vi "MailWake.vi"() -> ()   [LabVIEW 2012]
panel:
  out "Messages:":string[][](table)
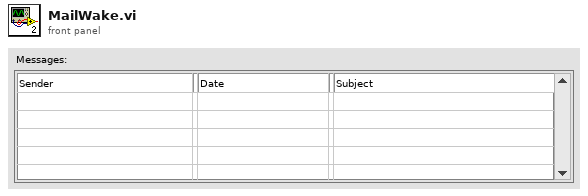
[diagram p1: front panel]
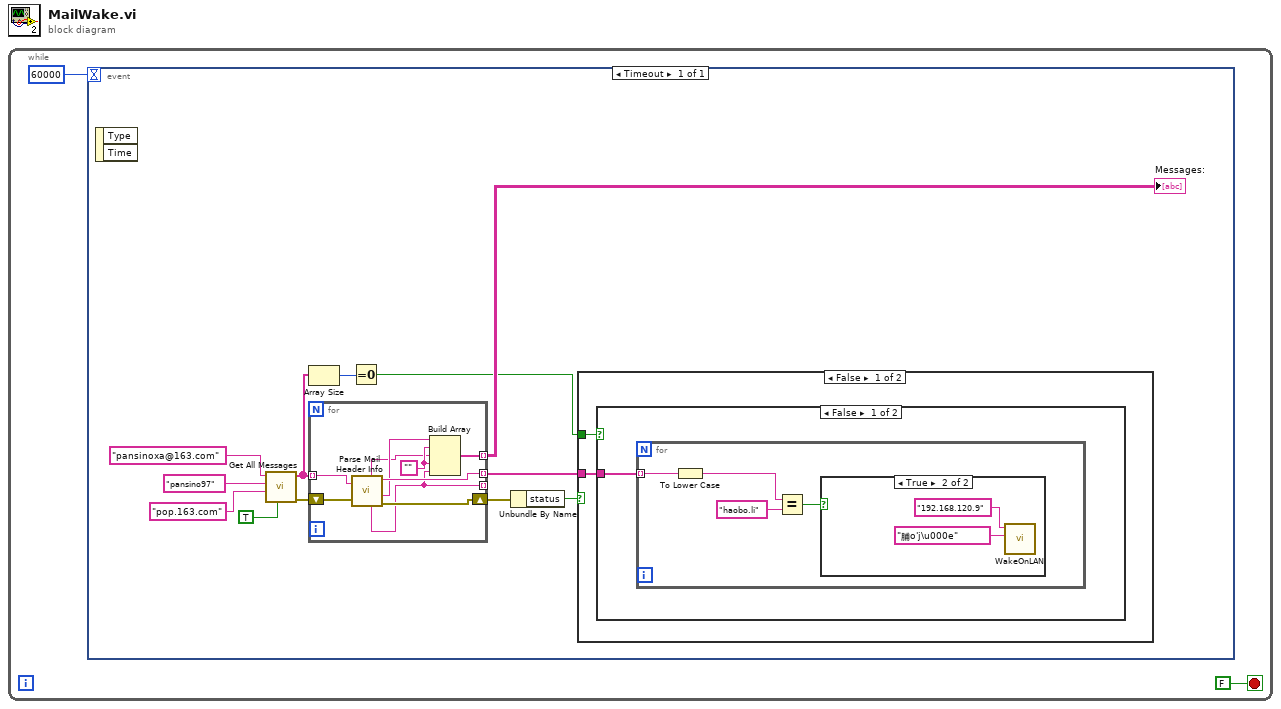
[diagram p0: block diagram]
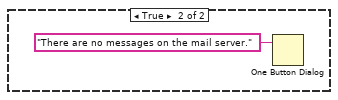
[diagram p3: hidden frame]
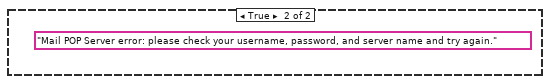
[diagram p4: hidden frame]
diagram:
  n1 = while {
    stop <- FALSE stop-if-true
    n2 = event shown="[0] Timeout" {
      selector: _ -> [_]
      dyn-events: _ -> [_]
      timeout: 60000 -> [_]
      event Timeout {
        n3 = event-data() -> ()  [unwired: 1 in, 2 out]
        n4 = call "Get All Messages.vi"("delete from server (Y)?"=TRUE, "POP server name/IP"="pop.163.com" ("POP server:"), "password"="pansino97" ("Password:"), "username"="pansinoxa@163.com" ("Username:")) -> ("error out"=w10:errorcluster, "message array"=w5:string[])  [unwired: 4 in, 1 out]
        n5 = Array Size(array=w5) -> (size(s)=w4:i32)
        n6 = for {
          tunnel: w5 -> [w33] mode=indexing
          shift-right: [w31] -> w8
          shift-left: w10 -> [w32]
          tunnel: [w30] -> w9 mode=indexing
          tunnel: [w28] -> w6 mode=indexing
          tunnel: [w25] -> _ mode=indexing
          w27 = ""
          n7 = call "Parse Mail Header Info.vi"("Message Content"=w33, "error in (no error)"=w32) -> ("Date"=w26:string, "Subject"=w25:string, "Message Content out"=w30:string, "From"=w29:string, "error out"=w31:errorcluster)  [unwired: 1 out]
          n8 = Build Array(w29, w27, w26, w27, w25) -> (w28:string[])
        }
        "Messages:" <- w6
        n9 = Equal To 0?(x=w4) -> (x = 0?=w3:bool)
        n10 = Unbundle By Name(w8) -> ("status"=w7:bool)
        n11 = case shown="False" w7 {
          tunnel: w9 -> [w16 _]
          tunnel: w3 -> [w15 _]
          frame False {
            n12 = case shown="False" w15 {
              tunnel: w16 -> [w17 _]
              frame False {
                n13 = for {
                  tunnel: w17 -> [w21] mode=indexing
                  n14 = To Lower Case(string=w21) -> (all lower case string=w19:string)
                  n15 = Equal?(x=w19, y="haobo.li") -> (x = y?=w18:bool)
                  n16 = case shown="True" w18 {
                    frame False {
                    }
                    frame True {
                      n17 = call "WakeOnLAN.vi"("Mac Address"="脯o'j\u000e", "IP of the computer to control"="192.168.120.9") -> ()  [unwired: 10 in]
                    }
                  }
                }
              }
              frame True {
                n18 = One Button Dialog(message="There are no messages on the mail server.") -> ()  [unwired: 1 in, 1 out]
              }
            }
          }
          frame True {
            (unwired) "Mail POP Server error: please check your username, password, and server name and try again." ("message")
          }
        }
      }
    }
  }
